vi "unwrap data.vi"(10 "identifier":string, 11 "data to unwrap":string) -> (2 "unwrapped data":string, 3 "remaining string":string)   [LabVIEW 2013, in "TBM configuration.lvclass"]
doc: "Parses a dataset of the following form:\n<identifier>data to wrap</identifier>"
uses:
  TBM configuration.lvclass
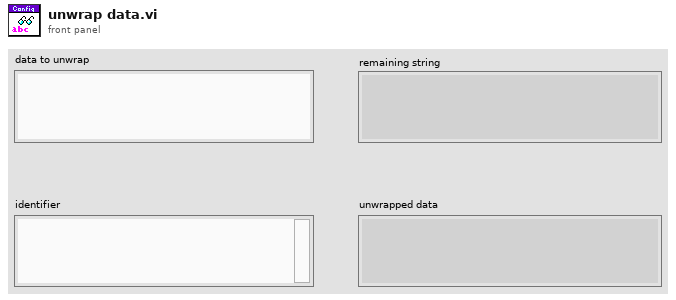
[diagram p1: front panel]
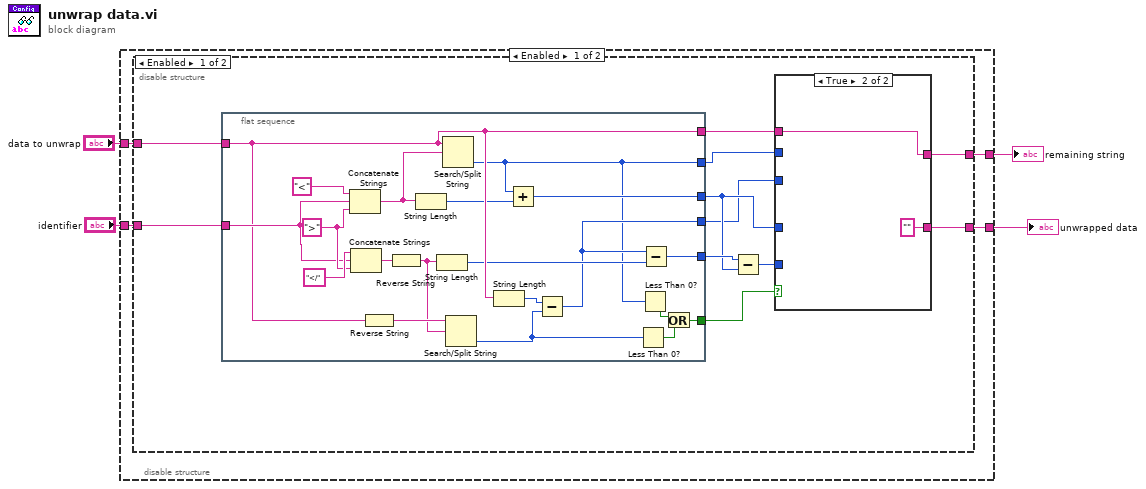
[diagram p0: block diagram]
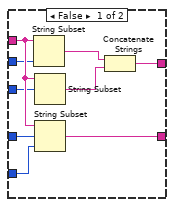
[diagram p2: hidden frame]
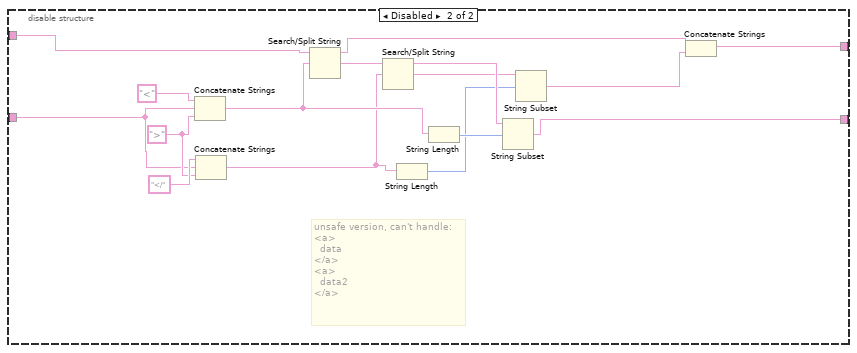
[diagram p3: hidden frame]
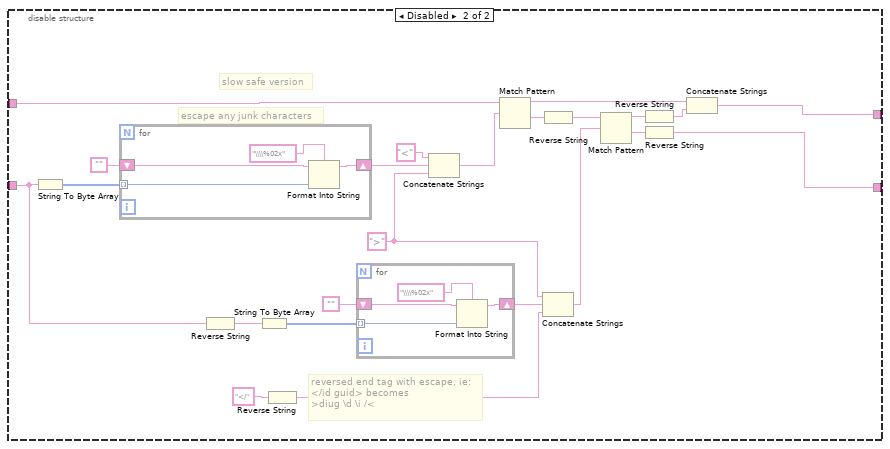
[diagram p4: hidden frame]
diagram:
  n1 = disable-structure shown="Enabled" {
    disable-tunnel: [w5 w89] -> w4
    disable-tunnel: "data to unwrap" -> [w8 w88]
    disable-tunnel: [w6 w87] -> w2
    disable-tunnel: "identifier" -> [w7 w86]
    frame Enabled {
      n2 = disable-structure shown="Enabled" {
        disable-tunnel: w7 -> [w19 w53]
        disable-tunnel: w8 -> [w18 w54]
        disable-tunnel: [w17 w51] -> w6
        disable-tunnel: [w16 w52] -> w5
        frame Enabled {
          n3 = flat-sequence {
            tunnel: w19 -> [w47]
            tunnel: w18 -> [w43]
            tunnel: [w34] -> w14
            tunnel: [w43] -> w15
            tunnel: [w40] -> w12
            tunnel: [w37] -> w13
            tunnel: [w36] -> w10
            tunnel: [w31] -> w9
            frame #0 {
              w48 = ">" ("string")
              n4 = Concatenate Strings("<" ("string"), w47, w48) -> (w42:string)
              n5 = Concatenate Strings("</" ("string"), w47, w48) -> (w46:string)
              n6 = Reverse String(1:w43) -> (0:w45:string)
              n7 = Reverse String(1:w46) -> (0:w39:string)
              n8 = String Length(string=w42) -> (length=w41:i32)
              n9 = String Length(string=w39) -> (length=w38:i32)
              n10 = Search/Split String(string=w43, search string/char (-)=w42) -> (offset of match=w34:i32)  [unwired: 1 in, 2 out]
              n11 = Search/Split String(string=w45, search string/char (-)=w39) -> (offset of match=w35:i32)  [unwired: 1 in, 2 out]
              n12 = String Length(string=w43) -> (length=w44:i32)
              n13 = Add(x=w34, y=w41) -> (x+y=w40:i32)
              n14 = Subtract(x=w44, y=w35) -> (x-y=w36:i32)
              n15 = Less Than 0?(x=w35) -> (x < 0?=w32:bool)
              n16 = Less Than 0?(x=w34) -> (x < 0?=w33:bool)
              n17 = Subtract(x=w36, y=w38) -> (x-y=w37:i32)
              n18 = Or(x=w33, y=w32) -> (x .or. y?=w31:bool)
            }
          }
          n19 = Subtract(x=w13, y=w12) -> (x-y=w11:i32)
          n20 = case shown="True" w9 {
            tunnel: [w28 w30] -> w17
            tunnel: [w27 "" ("data to unwrap")] -> w16
            tunnel: w15 -> [w24 w30]
            tunnel: w14 -> [w23 _]
            tunnel: w12 -> [w22 _]
            tunnel: w11 -> [w21 _]
            tunnel: w10 -> [w20 _]
            frame False {
              n21 = String Subset(string=w24, length (rest)=w23) -> (substring=w26:string)  [unwired: 1 in]
              n22 = String Subset(string=w24, offset (0)=w20) -> (substring=w25:string)  [unwired: 1 in]
              n23 = String Subset(string=w24, offset (0)=w22, length (rest)=w21) -> (substring=w27:string)
              n24 = Concatenate Strings(w26, w25) -> (w28:string)
            }
            frame True {
            }
          }
        }
        frame Disabled {
          w64 = ">" ("string")
          # "unsafe version, can't handle:\n<a>\n  data\n</a>\n<a>\n  data2\n</a>"
          n25 = Concatenate Strings("<" ("string"), w53, w64) -> (w59:string)
          n26 = Concatenate Strings("</" ("string"), w53, w64) -> (w56:string)
          n27 = Search/Split String(string=w54, search string/char (-)=w59) -> (substring before match=w62:string, match + rest of string=w63:string)  [unwired: 1 in, 1 out]
          n28 = Search/Split String(string=w63, search string/char (-)=w56) -> (substring before match=w61:string, match + rest of string=w58:string)  [unwired: 1 in, 1 out]
          n29 = String Length(string=w56) -> (length=w55:i32)
          n30 = String Length(string=w59) -> (length=w60:i32)
          n31 = String Subset(string=w61, offset (0)=w60) -> (substring=w52:string)  [unwired: 1 in]
          n32 = String Subset(string=w58, offset (0)=w55) -> (substring=w57:string)  [unwired: 1 in]
          n33 = Concatenate Strings(w62, w57) -> (w51:string)
        }
      }
    }
    frame Disabled {
      w79 = ">" ("string")
      # "slow safe version"
      # "escape any junk characters"
      # "reversed end tag with escape, ie:\n</id guid> becomes\n>diug \\d \\i /<"
      n34 = String To Byte Array(string=w86) -> (unsigned byte array=w84:u8[])
      n35 = for {
        tunnel: w84 -> [w97] mode=indexing
        shift-right: [w96] -> w80
        shift-left: "" -> [w95]
        n36 = Format Into String(format string="\\\\%02x", initial string=w95, w97) -> (resulting string=w96:string)  [unwired: 1 in, 1 out]
      }
      n37 = Reverse String(1:w86) -> (0:w75:string)
      n38 = String To Byte Array(string=w75) -> (unsigned byte array=w76:u8[])
      n39 = Reverse String(1:"</" ("string")) -> (0:w73:string)
      n40 = for {
        tunnel: w76 -> [w93] mode=indexing
        shift-right: [w92] -> w74
        shift-left: "" -> [w91]
        n41 = Format Into String(format string="\\\\%02x", initial string=w91, w93) -> (resulting string=w92:string)  [unwired: 1 in, 1 out]
      }
      n42 = Concatenate Strings("<" ("string"), w80, w79) -> (w82:string)
      n43 = Match Pattern(string=w88, regular expression=w82) -> (before substring=w69:string, after substring=w72:string)  [unwired: 1 in, 2 out]
      n44 = Reverse String(1:w72) -> (0:w71:string)
      n45 = Concatenate Strings(w79, w74, w73) -> (w81:string)
      n46 = Match Pattern(string=w71, regular expression=w81) -> (before substring=w68:string, after substring=w70:string)  [unwired: 1 in, 2 out]
      n47 = Reverse String(1:w68) -> (0:w67:string)
      n48 = Reverse String(1:w70) -> (0:w89:string)
      n49 = Concatenate Strings(w69, w67) -> (w87:string)
    }
  }
  "unwrapped data" <- w4
  "remaining string" <- w2
